vi "get id.vi"(8 "error in (no error)":errorcluster, 11 "img in":refnum<class "img.lvclass">) -> (0 "error out":errorcluster, 2 "id":i32, 3 "img out":refnum<class "img.lvclass">)   [LabVIEW 2013, in "DatenKlassen.lvlib" / "img.lvclass"]
uses:
  img.lvclass
  img.lvclass/img.ctl
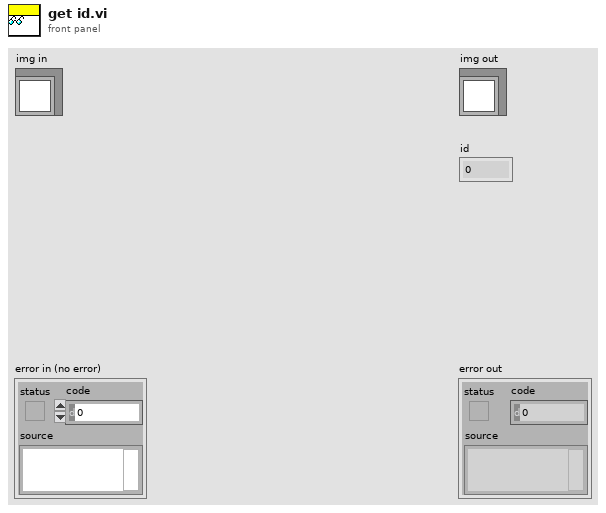
[diagram p1: front panel]
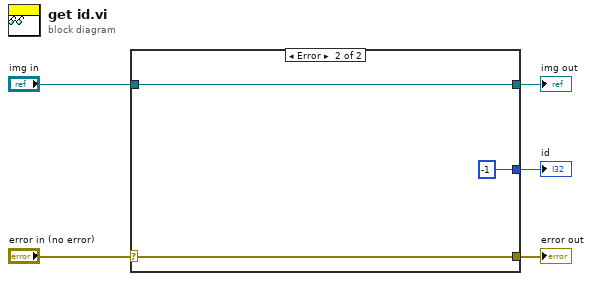
[diagram p0: block diagram]
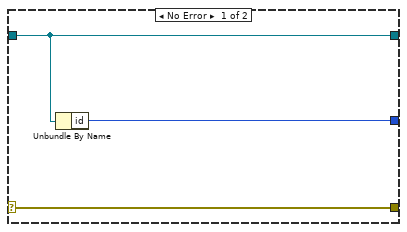
[diagram p2: hidden frame]
diagram:
  n1 = case shown="Error" "error in (no error)" {
    selector: "error in (no error)" -> [w8 w10]
    tunnel: [w8 w10] -> w4
    tunnel: [w7 w11] -> w2
    tunnel: "img in" -> [w7 w11]
    tunnel: [w6 -1 ("id")] -> w1
    frame No Error {
      n2 = Unbundle By Name(w7) -> ("id"=w6:i32)
    }
    frame Error {
    }
  }
  "error out" <- w4
  "img out" <- w2
  "id" <- w1
